vi "APPLICATION MAIN.vi"() -> ()   [LabVIEW 2015]
uses:
  <vilib>/Espotel/IoT Foundation/IoTF/CTLs/IoTF Application Subscription.ctl
  <vilib>/Espotel/IoT Foundation/MQTT/Public CTLs/MQTT QoS.ctl
  <vilib>/Espotel/IoT Foundation/IoTF/CTLs/IoTF Application Credentials.ctl
  Sources/Sensors Data.ctl
  <vilib>/Espotel/IoT Foundation/IoTF/CTLs/IoTF Message.ctl
  Sources/Relay State.ctl
  <vilib>/Espotel/IoT Foundation/IoTF/CTLs/IoTF Device Specifier.ctl
  <vilib>/Espotel/IoT Foundation/IoTF/IoTF Library.lvlib
  <vilib>/Espotel/IoT Foundation/MQTT/MQTT Library.lvlib
panel:
  out "Obstacle":bool
  out "Yeah Magnets!!":bool
  out "App Working":bool
  out "Fire Alarm":bool
  out "Connected":bool
  out "Sound":sgl[](graph)
  out "Accelerometer":cluster{"X":i8, "Y":i8, "Z":i8}(graph)
  in  "Process Stop Button":bool
  # "App"
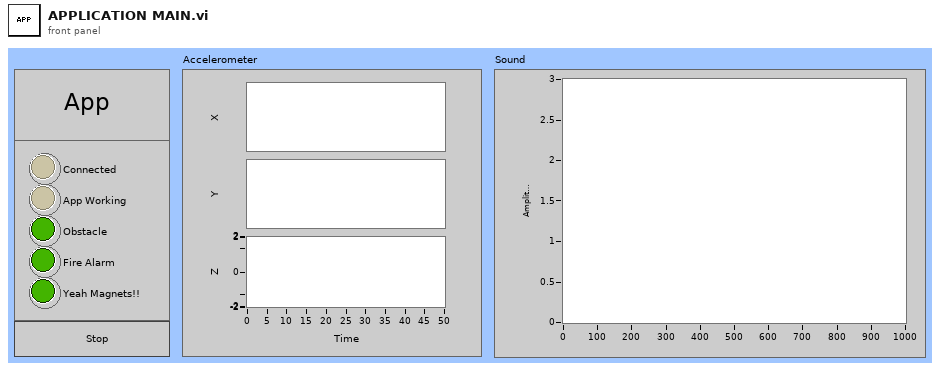
[diagram p1: front panel]
types:
  T1 = typedef "IoTF Library.lvlib/IoTF Application Credentials.ctl" = cluster{"Organization ID":string, "Application ID":string, "API Key":string, "Auth-token":string}
  T2 = typedef "IoTF Library.lvlib/IoTF Application Subscription.ctl" = cluster{"Subscription":string, "Device Type":string, "Device ID":string, "QoS":T3}
  T3 = typedef "MQTT Library.lvlib/MQTT QoS.ctl" = enum16{"At most once", "At least once", "Exactly once"}
  T4 = typedef "Sensors Data.ctl" = cluster{"X":i8, "Y":i8, "Z":i8, "flame":bool, "magnet":bool, "obstacle":bool, "sound":sgl[]}
  T5 = typedef "IoTF Library.lvlib/IoTF Device Specifier.ctl" = cluster{"Device Type":string, "Device ID":string}
  T6 = typedef "Relay State.ctl" = cluster{"Relay State":bool}
  T7 = typedef "IoTF Library.lvlib/IoTF Message.ctl" = cluster{"Message ID":string, "JSON object":string, "QoS":T3, "Include timestamp?":bool, "Custom JSON payload?":bool}
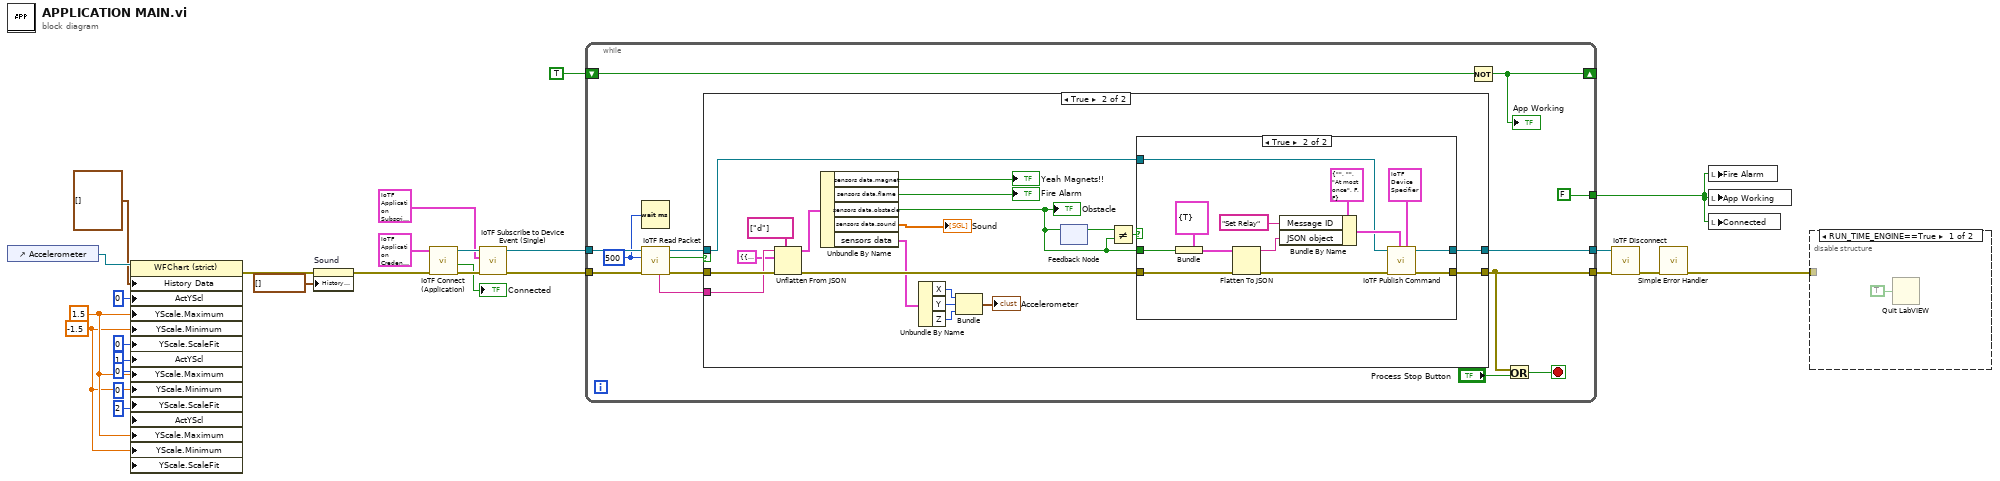
[diagram p0: block diagram]
diagram:
  w10 = -1.5 ("Y Scale.Range:Minimum")
  w11 = 1.5 ("Y Scale.Range:Maximum")
  n1 = control-ref of="Accelerometer"() -> (w7:refnum<vi>)
  n2 = property on="Property Node" class="WFChart (strict)"(reference=w7, "History Data"=cluster{"X":i8, "Y":i8, "Z":i8}[] [], "ActYScl"=0 ("Active Y Scale"), "YScale.Maximum"=w11, "YScale.Minimum"=w10, "YScale.ScaleFit"=u8 0 ("Y Scale.Scale Fit"), "ActYScl"=1 ("Active Y Scale"), "YScale.Maximum"=w11, "YScale.Minimum"=w10, "YScale.ScaleFit"=u8 0 ("Y Scale.Scale Fit"), "ActYScl"=2 ("Active Y Scale"), "YScale.Maximum"=w11, "YScale.Minimum"=w10, "YScale.ScaleFit"=u8 0 ("Y Scale.Scale Fit")) -> (error out=w5:errorcluster)  [unwired: 1 in, 1 out]
  n3 = property on="Sound" class="WFChart (strict)"(error in=w5, "History Data"=waveform(sgl)[] []) -> (error out=w4:errorcluster)  [unwired: 1 in, 1 out]
  n4 = call <vilib>:"IoTF Connect (Application).vi"("Error in (no error)"=w4, "IoTF Application Credentials"=T1 {"Organization ID"="hlkhwz", "Application ID"="LabVIEW_App", "API Key"="a-hlkhwz-u85cgcclrk", "Auth-token"="Jh0jqp9ak+9xFl(96!"}) -> ("Error out"=w25:errorcluster, "Connection accepted?"=→"Connected":bool, "Connection ID out"=w26:refnum<k5>)  [unwired: 5 in, 2 out]
  n5 = call <vilib>:"IoTF Subscribe to Device Event (Single).vi"("Error in (no error)"=w25, "Subscription"=T2 {"Subscription"="Sensors Data", "Device Type"="LabVIEW_Minion", "Device ID"="Minion-00", "QoS"=enum."At most once"}, "Connection ID in"=w26) -> ("Error out"=w20:errorcluster, "Connection ID out"=w21:refnum<k5>)  [unwired: 5 in, 2 out]
  n6 = while {
    tunnel: w21 -> [w40]
    tunnel: w20 -> [w39]
    tunnel: [w33] -> w19
    tunnel: [w32] -> w18
    shift-right: [w28] -> _
    shift-left: TRUE ("Relay State") -> [w29]
    tunnel: [FALSE ("Relay State")] -> w2
    stop <- w30 stop-if-true
    w38 = 500 ("Timeout (10000ms)")
    n7 = Wait (ms)(milliseconds to wait=w38) -> ()  [unwired: 1 out]
    n8 = call <vilib>:"IoTF Read Packet.vi"("Error in (no error)"=w39, "Timeout (10000ms)"=w38, "Connection ID in"=w40) -> ("Error out"=w35:errorcluster, "Packet Arrived?"=w37:bool, "Connection ID out"=w36:refnum<k5>, "Message"=w34:string)  [unwired: 4 in, 1 out]
    n9 = case shown="True" w37 {
      tunnel: w36 -> [w42 w58]
      tunnel: w35 -> [w41 w62]
      tunnel: w34 -> [_ w61]
      tunnel: [w42 w57] -> w33
      tunnel: [w41 w56] -> w32
      frame False {
      }
      frame True {
        n10 = Unflatten From JSON(path=string[] ["d"], JSON string=w61, type and defaults=cluster{"sensors data":T4} {"sensors data"={"X"=0, "Y"=0, "Z"=0, "flame"=TRUE, "magnet"=TRUE, "obstacle"=FALSE, "sound"=[]}}, error in (no error)=w62) -> (value=w55:cluster{"sensors data":T4}, error out=w59:errorcluster)  [unwired: 3 in]
        n11 = Unbundle By Name(w55) -> ("sensors data.magnet"=→"Yeah Magnets!!":bool, "sensors data.flame"=→"Fire Alarm":bool, "sensors data.obstacle"=w49:bool, "sensors data.sound"=→"Sound":sgl[], "sensors data"=w47:T4)
        "Obstacle" <- w49
        n12 = Unbundle By Name(w47) -> ("X"=w46:i8, "Y"=w45:i8, "Z"=w44:i8)
        n13 = Bundle("X"=w46, "Y"=w45, "Z"=w44) -> (→"Accelerometer":cluster{"X":i8, "Y":i8, "Z":i8})  [unwired: 1 in]
        n14 = feedback #1() -> (w54:bool)  [unwired: 1 in]
        n15 = feedback-in #1(w49) -> ()
        n16 = Not Equal?(x=w54, y=w49) -> (x != y?=w53:bool)
        n17 = case shown="True" w53 {
          tunnel: w59 -> [w64 w69]
          tunnel: [w64 w68] -> w56
          tunnel: w58 -> [w63 w67]
          tunnel: [w63 w66] -> w57
          tunnel: w49 -> [_ w65]
          frame False {
          }
          frame True {
            n18 = Bundle(cluster=T6 {"Relay State"=TRUE} ("d"), "Relay State"=w65) -> (w72:T6)
            n19 = Flatten To JSON(anything=w72, error in (no error)=w69) -> (JSON string=w75:string, 11:w76:errorcluster)  [unwired: 1 in]
            n20 = Bundle By Name(cluster=T7 {"Message ID"="", "JSON object"="", "QoS"=enum."At most once", "Include timestamp?"=FALSE, "Custom JSON payload?"=FALSE} ("IoTF Message"), "Message ID"="Set Relay", "JSON object"=w75) -> (w74:T7)
            n21 = call <vilib>:"IoTF Publish Command.vi"("Device Specifier"=T5 {"Device Type"="LabVIEW_Minion", "Device ID"="Minion-00"}, "IoTF Message"=w74, "Error in (no error)"=w76, "Connection ID in"=w67) -> ("Error out"=w68:errorcluster, "Connection ID out"=w66:refnum<k5>)  [unwired: 5 in, 1 out]
          }
        }
      }
    }
    n22 = Not(x=w29) -> (.not. x?=w28:bool)
    "App Working" <- w28
    n23 = Or(x=w32, y="Process Stop Button") -> (x .or. y?=w30:bool)
  }
  n24 = call <vilib>:"IoTF Disconnect.vi"("Error in (no error)"=w18, "Connection ID in"=w19) -> ("Error out"=w16:errorcluster)  [unwired: 8 in, 1 out]
  n25 = call <vilib>:"Simple Error Handler.vi"("error in (no error)"=w16) -> ("error out"=w1:errorcluster)  [unwired: 4 in, 4 out]
  n26 = local write "Fire Alarm"(w2) -> ()
  n27 = local write "App Working"(w2) -> ()
  n28 = local write "Connected"(w2) -> ()
  n29 = disable-structure shown="RUN_TIME_ENGINE==True" {
    disable-tunnel: w1 -> [_ _]
    frame condition #0 {
      n30 = Quit LabVIEW(quit? (T)=TRUE) -> ()
    }
    frame condition #1 (active) {
    }
  }
